vi "Get Number Amp.vi"(11 "amp":i32) -> (2 "function return":u32, 3 "amp out":i32)   [LabVIEW 2018, in "AndorSDK.lvlib"]
doc: "EXPNETTYPE unsigned int WINAPI GetNumberAmp(int * amp);"
uses:
  AndorSDK.lvlib
  ATMCD32D.dll
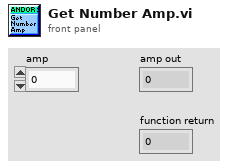
[diagram p1: front panel]
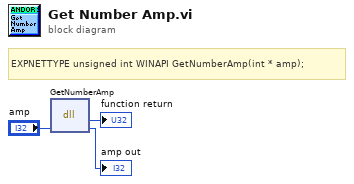
[diagram p0: block diagram]
diagram:
  # "EXPNETTYPE unsigned int WINAPI GetNumberAmp(int * amp);"
  n1 = dll-call lib="PTH2babs E\nPersönliches02 - Arbeit03-HiwijobsLabviewCodelibANDOR\tAndor SDK\nATMCD32D.*" fn="GetNumberAmp"("amp"="amp") -> (→"function return":u32, "amp"=→"amp out":i32)  [unwired: 3 in, 2 out]
